vi "Get Data from TSM Global.vi"(8 "error in (no error)":errorcluster, 10 "LookUp String":string="409.75M_Freq", 11 "Semiconductor Module Context":T1) -> (0 "error out":errorcluster, 3 "Look Up Value":dbl)   [LabVIEW 2014]
uses:
  <vilib>/NI_TestStand_SemiconductorModule/NI_TestStand_Semiconductor_Module.lvlibp/PinMap/General/SemiconductorModuleContext.ctl
  <vilib>/NI_TestStand_SemiconductorModule/NI_TestStand_Semiconductor_Module.lvlibp
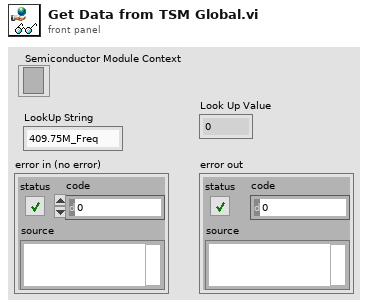
[diagram p1: front panel]
types:
  T1 = typedef "NI_TestStand_Semiconductor_Module.lvlibp/SemiconductorModuleContext.ctl" = refnum<k7>
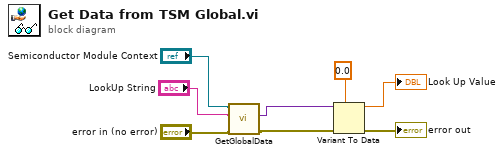
[diagram p0: block diagram]
diagram:
  n1 = call <vilib>:"GetGlobalData.vi"("error in (no error)"="error in (no error)", "Data Id"="LookUp String", "Semiconductor Module Context"="Semiconductor Module Context") -> ("error out"=w4:errorcluster, "Data"=w1:variant)  [unwired: 6 in, 1 out]
  n2 = Variant To Data(error in=w4, type=0.0 ("power"), Variant=w1) -> (data=→"Look Up Value":dbl, error out=→"error out":errorcluster)
